vi "Drive Controller.vi"(8 "error in":errorcluster) -> ()   [LabVIEW 2020]
doc: "This VI executes continuously carrying out the current operation and responding to updates or new operation requests. It will often contain the timing or control code that is difficult to place directly in TeleOp. This VI generally opens all sensors and motors and isolates the rest of the robot code from knowing implementation details of how the operations are carried out."
uses:
  swerve/ctl/Pod Setpoints.ctl
  Drive Setpoints.ctl
  Drive Operations.ctl
  Robot Velocities.ctl
  <vilib>/Rock Robotics/WPI/ThirdParty/Phoenix-LabVIEW/Motor Controller/Controls/CTRE_Phoenix_MotorControl_ControlMode.ctl
  <vilib>/Analysis/coordinate.llb/Angle Range (Degree).ctl
  <vilib>/Analysis/coordinate.llb/Angle Units.ctl
  <vilib>/Analysis/coordinate.llb/Wrap Angle (array).vi
  <vilib>/Rock Robotics/Network Tables/NT Write Numeric Array.vi
  <vilib>/Analysis/NI_AAL_Angle.lvlib
panel:
  in  "Pod Setpoints (ft/s and deg)":T1
  out "CANCoder Angles":T2
  out "Calibration Error":errorcluster
  out "Initial Error":errorcluster
  out "Current\nCmd":string
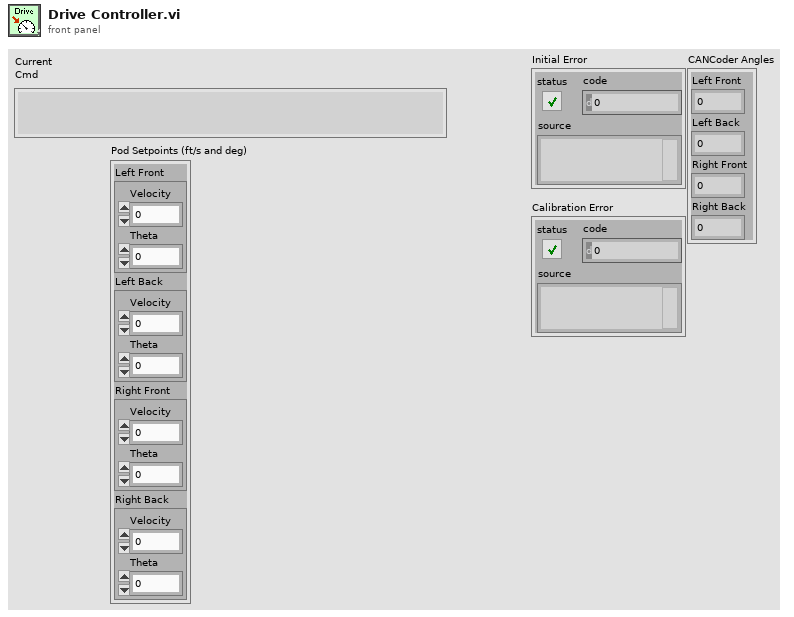
[diagram p1: front panel]
types:
  T1 = typedef "Pod Setpoints.ctl" = cluster{"Left Front":cluster{"Velocity":dbl, "Theta":dbl}, "Left Back":cluster{"Velocity":dbl, "Theta":dbl}, "Right Front":cluster{"Velocity":dbl, "Theta":dbl}, "Right Back":cluster{"Velocity":dbl, "Theta":dbl}}
  T2 = cluster{"Left Front":dbl, "Left Back":dbl, "Right Front":dbl, "Right Back":dbl}
  T3 = cluster{"LF radius":dbl[], "LB radius":dbl[], "RF radius":dbl[], "RB radius":dbl[]}
  T4 = cluster{"LF ID":u8, "LB ID":u8, "RF ID":u8, "RB ID":u8}
  T5 = typedef "Drive Setpoints.ctl" = cluster{"Operation":T6, "Robot Velocities":T7, "Field Centric?":bool, "Auto Velocities":T7[]}
  T6 = typedef "Drive Operations.ctl" = enum16{"Reserve", "Read Current", "Immediate", "Calibrate", "Reset Pods", "Auto"}
  T7 = typedef "Robot Velocities.ctl" = cluster{"vx":dbl, "vy":dbl, "w":dbl}
  T8 = typedef "Swerve Motors.ctl" = cluster{"Drive Motors":T9, "Steering Motors":T9}
  T9 = typedef "4 Motor Set.ctl" = cluster{"Left Front":T10, "Left Back":T10, "Right Front":T10, "Right Back":T10}
  T10 = typedef "WPI_MotorControlDeviceRef.ctl" = cluster{"DeviceStatus":errorcluster, "Type":T11, "PWM":cluster{"PWM Channel":T12, "DeadBand":T13}, "CAN":cluster{"Device Number":u8, "SetOutput VI Ref":variant, "GetOutput VI Ref":variant, "Enable VI Ref":variant, "Disable VI Ref":variant, "Data":variant}, "Invert":bool, "DIO PWM":cluster{"PWM \"Enable\" Channel":T12, "DIOChannel":T14, "PWM Rate":dbl}}
  T11 = typedef "WPI_MotorControlType.ctl" = enum16{"PWM", "CAN", "DIO PWM"}
  T12 = typedef "FPGA_DIOPWMChannel.ctl" = enum8{"PWM 0", "PWM 1", "PWM 2", "PWM 3", "PWM 4", "PWM 5", "PWM 6", "PWM 7", "PWM 8", "PWM 9", "PWM MXP 0", "PWM MXP 1", "PWM MXP 2", "PWM MXP 3", "PWM MXP 4", "PWM MXP 5", "PWM MXP 6", "PWM MXP 7", "PWM MXP 8", "PWM MXP 9", "Invalid"}
  T13 = typedef "WPI_PWMDeadband.ctl" = cluster{"Name":string, "maxPositivePwm":i32, "minPositivePwm":i32, "centerPwm":i32, "maxNegativePwm":i32, "minNegativePwm":i32, "angularRange":u16}
  T14 = typedef "FPGA_DIOChannel.ctl" = enum8{"DIO 0", "DIO 1", "DIO 2", "DIO 3", "DIO 4", "DIO 5", "DIO 6", "DIO 7", "DIO 8", "DIO 9", "DIO MXP 0", "DIO MXP 1", "DIO MXP 2", "DIO MXP 3", "DIO MXP 4", "DIO MXP 5", "DIO MXP 6", "DIO MXP 7", "DIO MXP 8", "DIO MXP 9", "DIO MXP 10", "DIO MXP 11", "DIO MXP 12", "DIO MXP 13", "DIO MXP 14", "DIO MXP 15", "SPI Port CS1", "SPI Port CS2", "SPI Port CS3", "SPI Port MISO", "SPI Port MOSI", "Invalid"}
  T15 = typedef "Swerve CANCoders.ctl" = cluster{"Left Front":T16, "Left Back":T16, "Right Front":T16, "Right Back":T16}
  T16 = typedef "CTRE_Phoenix_CANcoder_DeviceRef.ctl" = cluster{"DeviceStatus":errorcluster, "Device Number":u8, "Handle":u64, "UsageFrame":u32, "Library Path":path}
  T17 = typedef "Command Status Info.ctl" = cluster{"Name":string, "Status":T18, "notifier out":T19}
  T18 = typedef "Completion Status.ctl" = enum16{"Successful", "Aborted", "Incomplete"}
  T19 = typedef "Completion Notifier.ctl" = refnum<notifier>
  T20 = cluster{"SubSystem Data":T5, cluster{"Start Time (ms)":u32, "Iterations":i32}, cluster{"Command Info":T17, "Description":string, "Default Command":T5, "queue out":refnum<queue>, "Subsystem Name":string}}
  T21 = typedef "CTRE_PigeonIMU_DeviceRef.ctl" = cluster{"DeviceStatus":errorcluster, "Device Number":u8, "Type":T22, "Device ID":u32, "Handle":u64, "UsageFrame":u32, "Library Path":path}
  T22 = typedef "CTRE_PigeonIMU_ConnectionType.ctl" = u32
  T23 = typedef "CTRE_Phoenix_MotorControl_ControlMode.ctl" = u16
  T24 = cluster{"SubSystem Data":T5, cluster{"Start Time (ms)":u32, "Iterations":i32}, "Default Command Arguments":cluster{"Command Info":T17, "Description":string, "Default Command":T5, "queue out":refnum<queue>, "Subsystem Name":string}}
  T25 = typedef "NI_AAL_Angle.lvlib/Angle Units.ctl" = i32
  T26 = typedef "NI_AAL_Angle.lvlib/Angle Range (Degree).ctl" = u16
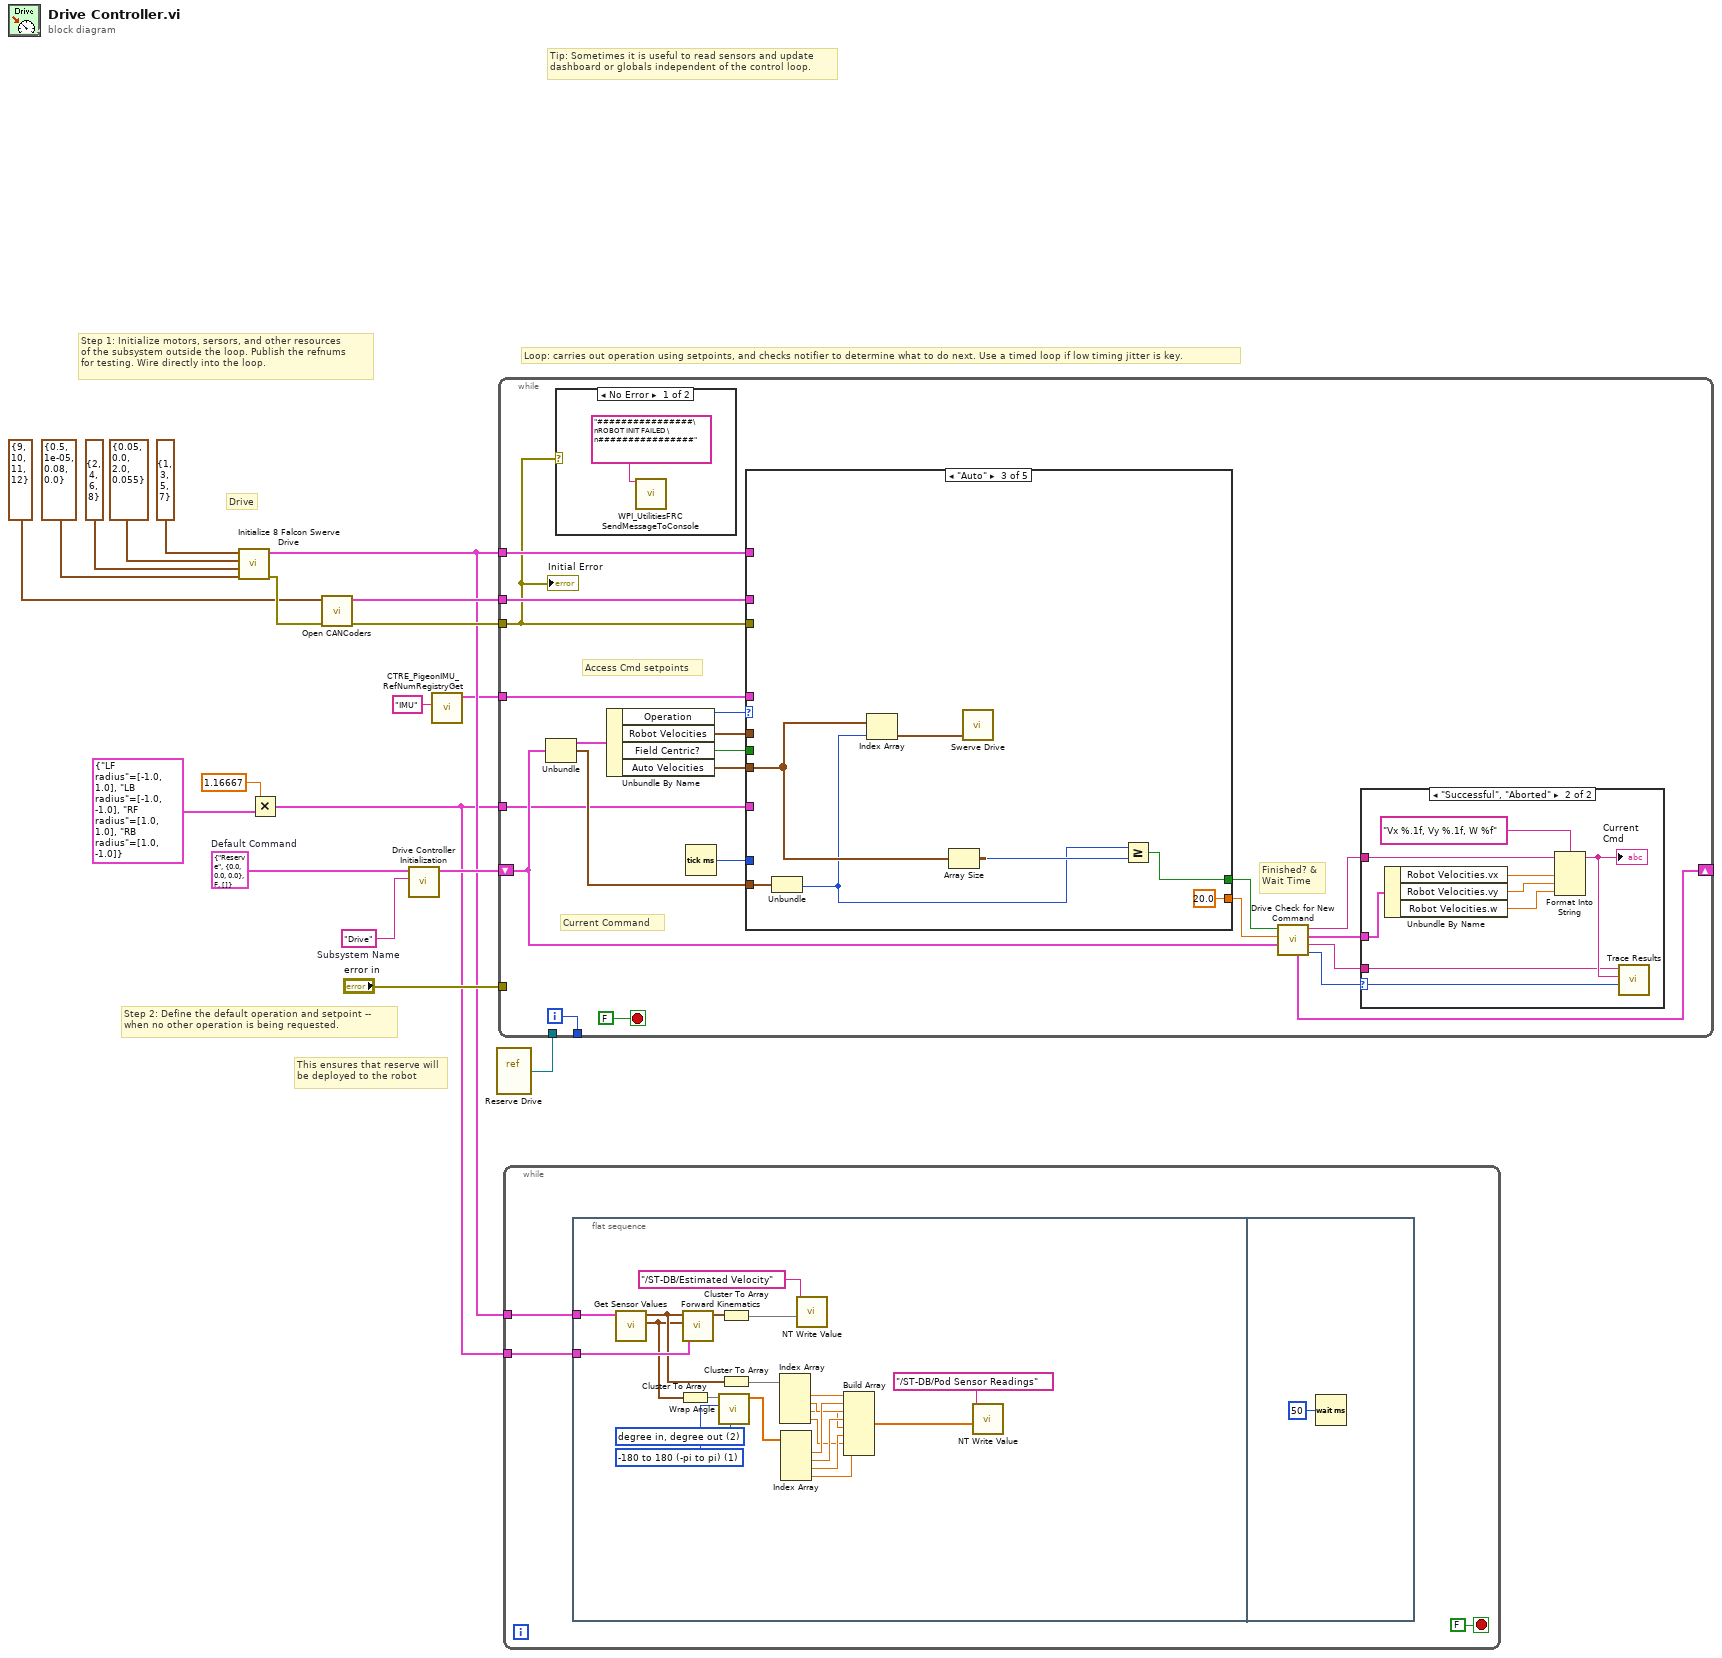
[diagram p0: block diagram]
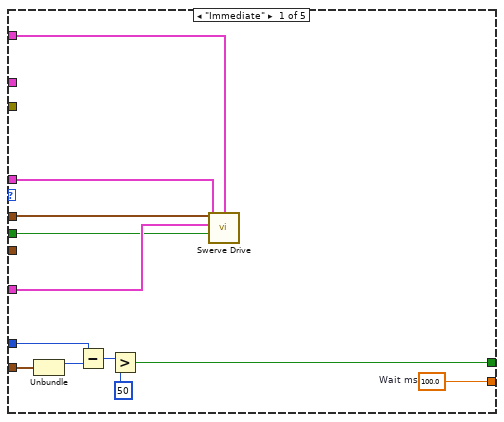
[diagram p4: hidden frame]
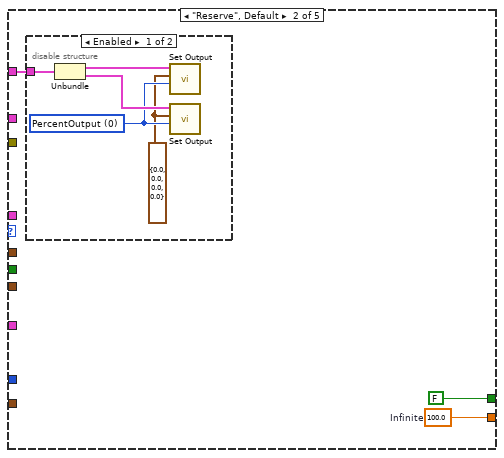
[diagram p5: hidden frame]
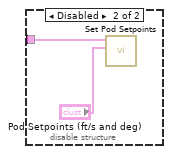
[diagram p6: hidden frame]
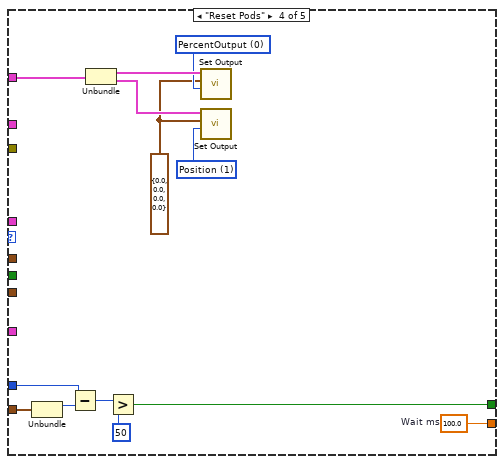
[diagram p7: hidden frame]
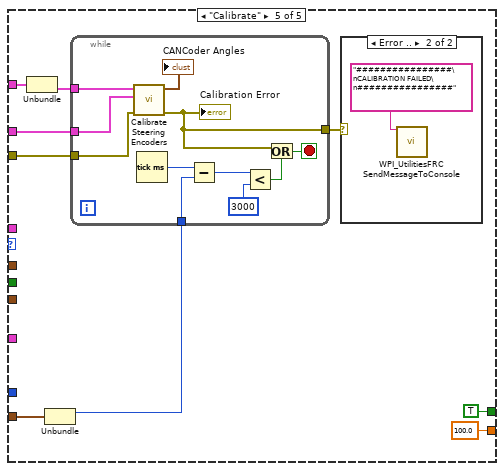
[diagram p8: hidden frame]
diagram:
  w15 = T5 {"Operation"=enum."Reserve", "Robot Velocities"={"vx"=0.0, "vy"=0.0, "w"=0.0}, "Field Centric?"=FALSE, "Auto Velocities"=[]}  # Default Command
  w19 = "Drive"  # Subsystem Name
  # "Drive"
  # "This ensures that reserve will\nbe deployed to the robot"
  # "Step 2: Define the default operation and setpoint --\nwhen no other operation is being requested."
  # "Step 1: Initialize motors, sersors, and other resources\nof the subsystem outside the loop. Publish the refnums\nfor testing. Wire directly into the loop."
  # "Loop: carries out operation using setpoints, and checks notifier to determine what to do next. Use a timed loop if low timing jitter is key."
  # "Tip: Sometimes it is useful to read sensors and update\ndashboard or globals independent of the control loop."
  n1 = call "Initialize 8 Falcon Swerve Drive.vi"("Steer PIDF"=cluster{"P":dbl, "I":dbl, "D":dbl, "F":dbl} {"P"=0.5, "I"=1e-05, "D"=0.08, "F"=0.0} ("PIDF"), "Steer CAN IDs"=T4 {"LF ID"=2, "LB ID"=4, "RF ID"=6, "RB ID"=8} ("Can IDs"), "Drive PIDF"=cluster{"P":dbl, "I":dbl, "D":dbl, "F":dbl} {"P"=0.05, "I"=0.0, "D"=2.0, "F"=0.055} ("PIDF"), "Drive CAN IDs"=T4 {"LF ID"=1, "LB ID"=3, "RF ID"=5, "RB ID"=7} ("Can IDs")) -> ("error out"=w10:errorcluster, "Motors"=w4:T8)  [unwired: 6 in]
  n2 = Multiply(x=1.16667, y=T3 {"LF radius"=[-1.0, 1.0], "LB radius"=[-1.0, -1.0], "RF radius"=[1.0, 1.0], "RB radius"=[1.0, -1.0]} ("Radii")) -> (x*y=w3:T3)
  n3 = call "Open CANCoders.vi"("error in"=w10, "CANCoder Can IDs"=T4 {"LF ID"=9, "LB ID"=10, "RF ID"=11, "RB ID"=12}) -> ("error out"=w7:errorcluster, "CANCoders"=w8:T15)  [unwired: 8 in]
  n4 = call "Drive Controller Initialization.vi"("Subsystem Name"=w19, "Default Command"=w15) -> ("Current Command"=w17:T20)  [unwired: 9 in]
  n5 = call <vilib>:"CTRE_PigeonIMU_RefNumRegistryGet.vi"("refnum name"="IMU") -> ("PigeonIMUDevRef"=w1:T21)  [unwired: 9 in, 1 out]
  n6 = vi-ref "Reserve Drive.vi"() -> (w16:refnum<vi>)
  n7 = while {
    shift-right: [w35] -> _
    shift-left: w17 -> [w28]
    tunnel: [w40] -> _
    tunnel: "error in" -> [_]
    tunnel: w16 -> [_]
    tunnel: w4 -> [w23]
    tunnel: w8 -> [w26]
    tunnel: w7 -> [w22]
    tunnel: w3 -> [w24]
    tunnel: w1 -> [w21]
    i -> [w40]
    stop <- FALSE stop-if-true
    # "Current Command"
    # "Access Cmd setpoints"
    # "Finished? &\nWait Time"
    n8 = Unbundle(w28) -> ("SubSystem Data"=w39:T5, w29:cluster{"Start Time (ms)":u32, "Iterations":i32})  [unwired: 1 out]
    n9 = case shown="No Error" w22 {
      frame No Error {
        n10 = call <vilib>:"WPI_UtilitiesFRC SendMessageToConsole.vi"("Message"="################\nROBOT INIT FAILED \n################") -> ()  [unwired: 14 in, 1 out]
      }
      frame Error {
      }
    }
    n11 = Unbundle By Name(w39) -> ("Operation"=w38:T6, "Robot Velocities"=w27:T7, "Field Centric?"=w25:bool, "Auto Velocities"=w20:T7[])
    n12 = Tick Count (ms)() -> (millisecond timer value=w37:u32)
    n13 = case shown="\"Auto\"" w38 {
      tunnel: [w63 w66 20.0 ("Infinite") w81 100.0 ("Infinite")] -> w34
      tunnel: [w55 FALSE ("ignore previous (F)") w75 w82 TRUE ("ignore previous (F)")] -> w33
      tunnel: w29 -> [w60 _ w80 w83 w96]
      tunnel: w37 -> [w59 _ _ w84 _]
      tunnel: w27 -> [w52 _ _ _ _]
      tunnel: w23 -> [w61 w64 _ w90 w99]
      tunnel: w26 -> [_ _ _ _ w102]
      tunnel: w22 -> [_ _ _ _ w100]
      tunnel: w25 -> [w54 _ _ _ _]
      tunnel: w24 -> [w62 _ _ _ _]
      tunnel: w21 -> [w53 _ _ _ _]
      tunnel: w20 -> [_ _ w77 _ _]
      frame "Immediate" {
        w63 = 100.0  # Wait ms
        n14 = Unbundle(w60) -> ("Start Time (ms)"=w58:u32)  [unwired: 1 out]
        n15 = Subtract(x=w59, y=w58) -> (x-y=w57:u32)
        n16 = Greater?(x=w57, y=u32 50) -> (0:w55:bool)
        n17 = call "Swerve Drive.vi"("Field Centric?"=w54, "Cluster"=w62, "Robot Velocities"=w52, "PigeonIMUDevRef"=w53, "Motors"=w61) -> ()  [unwired: 7 in]
      }
      frame "Reserve", Default {
        w66 = 100.0  # Infinite
        n18 = disable-structure shown="Enabled" {
          disable-tunnel: w64 -> [w71 w73]
          frame Enabled {
            w68 = T23 0 items=["PercentOutput"=0, "Position"=1, "Velocity"=2, "Current"=3, "Follower"=5, "MotionProfile"=6, "MotionMagic"=7, "MotionProfileArc"=10, "Disabled"=15] ("Control Mode")
            w67 = T2 {"Left Front"=0.0, "Left Back"=0.0, "Right Front"=0.0, "Right Back"=0.0} ("Setpoints")
            n19 = Unbundle(w71) -> ("Drive Motors"=w69:T9, "Steering Motors"=w70:T9)
            n20 = call "Set Output.vi"("Control Mode"=w68, "Setpoints"=w67, "Motors"=w69) -> ()  [unwired: 9 in]
            n21 = call "Set Output.vi"("Control Mode"=w68, "Setpoints"=w67, "Motors"=w70) -> ()  [unwired: 9 in]
          }
          frame Disabled {
            n22 = call "Set Pod Setpoints.vi"("Pod Setpoints (ft/s and deg)"="Pod Setpoints (ft/s and deg)", "Motors"=w73) -> ()  [unwired: 10 in]
          }
        }
      }
      frame "Auto" {
        n23 = Unbundle(w80) -> ("Iterations"=w74:i32)  [unwired: 1 out]
        n24 = Index Array(array=w77, index=w74) -> (element=w79:T7)
        n25 = Array Size(array=w77) -> (size(s)=w76:i32)
        n26 = call "Swerve Drive.vi"("Robot Velocities"=w79) -> ()  [unwired: 11 in]
        n27 = Greater Or Equal?(x=w74, y=w76) -> (x >= y?=w75:bool)
      }
      frame "Reset Pods" {
        w81 = 100.0  # Wait ms
        w88 = T2 {"Left Front"=0.0, "Left Back"=0.0, "Right Front"=0.0, "Right Back"=0.0} ("Setpoints")
        w89 = T23 0 items=["PercentOutput"=0, "Position"=1, "Velocity"=2, "Current"=3, "Follower"=5, "MotionProfile"=6, "MotionMagic"=7, "MotionProfileArc"=10, "Disabled"=15] ("Control Mode")
        w91 = T23 1 items=["PercentOutput"=0, "Position"=1, "Velocity"=2, "Current"=3, "Follower"=5, "MotionProfile"=6, "MotionMagic"=7, "MotionProfileArc"=10, "Disabled"=15] ("Control Mode")
        n28 = Unbundle(w83) -> ("Start Time (ms)"=w87:u32)  [unwired: 1 out]
        n29 = Subtract(x=w84, y=w87) -> (x-y=w86:u32)
        n30 = Unbundle(w90) -> ("Drive Motors"=w92:T9, "Steering Motors"=w93:T9)
        n31 = Greater?(x=w86, y=u32 50) -> (0:w82:bool)
        n32 = call "Set Output.vi"("Control Mode"=w89, "Setpoints"=w88, "Motors"=w92) -> ()  [unwired: 9 in]
        n33 = call "Set Output.vi"("Control Mode"=w91, "Setpoints"=w88, "Motors"=w93) -> ()  [unwired: 9 in]
      }
      frame "Calibrate" {
        n34 = Unbundle(w99) -> ("Steering Motors"=w98:T9)  [unwired: 1 out]
        n35 = Unbundle(w96) -> ("Start Time (ms)"=w95:u32)  [unwired: 1 out]
        n36 = while {
          tunnel: w102 -> [w114]
          tunnel: w100 -> [w113]
          tunnel: w98 -> [w112]
          tunnel: w95 -> [w109]
          tunnel: [w104] -> w94
          stop <- w110 stop-if-true
          n37 = call "Calibrate Steering Encoders.vi"("error in"=w113, "CANCoders"=w114, "Steering Motors"=w112) -> ("error out"=w104:errorcluster, "CANCoder Angles"=→"CANCoder Angles":T2)  [unwired: 7 in]
          "Calibration Error" <- w104
          n38 = Tick Count (ms)() -> (millisecond timer value=w108:u32)
          n39 = Subtract(x=w108, y=w109) -> (x-y=w107:u32)
          n40 = Less?(x=w107, y=u32 3000) -> (x < y?=w105:bool)
          n41 = Or(x=w104, y=w105) -> (x .or. y?=w110:bool)
        }
        n42 = case shown="Error .." w94 {
          frame No Error {
          }
          frame Error {
            n43 = call <vilib>:"WPI_UtilitiesFRC SendMessageToConsole.vi"("Message"="################\nCALIBRATION FAILED\n################") -> ()  [unwired: 14 in, 1 out]
          }
        }
      }
    }
    n44 = call "Drive Check for New Command.vi"("input cluster"=w28, "Wait time (ms)"=w34, "Finished?"=w33) -> ("Completion"=w36:T18, "Subsystem Name"=w30:string, "Current Command"=w31:T5, "Initial Trace String"=w32:string, "Next Command"=w35:T24)  [unwired: 4 in]
    n45 = case shown="\"Successful\", \"Aborted\"" w36 {
      selector: w36 -> [_ w51]
      tunnel: w32 -> [_ w46]
      tunnel: w31 -> [_ w47]
      tunnel: w30 -> [_ w43]
      frame "Incomplete", Default {
        # "Continuing current command"
      }
      frame "Successful", "Aborted" {
        # "Report and setup for next command"
        n46 = Unbundle By Name(w47) -> ("Robot Velocities.vx"=w49:dbl, "Robot Velocities.vy"=w50:dbl, "Robot Velocities.w"=w44:dbl)
        n47 = Format Into String(format string="Vx %.1f, Vy %.1f, W %f", initial string=w46, w49, w50, w44) -> (resulting string=w45:string)  [unwired: 1 in, 1 out]
        "Current\nCmd" <- w45
        n48 = call <vilib>:"Trace Results.vi"("Status of previous command"=w51, "Description"=w45, "Subsystem"=w43) -> ()  [unwired: 9 in]
      }
    }
    "Initial Error" <- w22
  }
  n49 = while {
    tunnel: w4 -> [w117]
    tunnel: w3 -> [w115]
    stop <- FALSE stop-if-true
    n50 = flat-sequence {
      tunnel: w117 -> [w139]
      tunnel: w115 -> [w138]
      frame #0 {
        w118 = T25 2 items=["radian in, radian out", "radian in, degree out", "degree in, degree out", "degree in, radian out"] ("angle units")
        w119 = T26 1 items=["none", "-180 to 180 (-pi to pi)", "0 to 360 (0 to 2pi)"] ("angle range")
        n51 = call "Get Sensor Values.vi"("Motors"=w139) -> ("Steer Angles (degrees)"=w122:T2, "Drive Velocities (ft/s)"=w133:T2)  [unwired: 7 in, 2 out]
        n52 = Cluster To Array(cluster=w122) -> (array=w121:dbl[])
        n53 = call "Forward Kinematics.vi"("Radii (ft)"=w138, "Steer Angles (degrees)"=w122, "Drive Velocities (ft/s)"=w133) -> ("Robot Velocities (ft and deg)/s"=w137:cluster{"vx":dbl, "vy":dbl, "w":dbl})  [unwired: 8 in]
        n54 = call-poly <vilib>:"Wrap Angle.vi"("angle units"=w118, "angle range"=w119, "Angle In"=w121) -> ("Angle Out"=w120:dbl[])  [unwired: 7 in, 1 out]
        n55 = Cluster To Array(cluster=w137) -> (array=w136:dbl[])
        n56 = Cluster To Array(cluster=w133) -> (array=w134:dbl[])
        n57 = Index Array(array=w134) -> (element #1=w131:dbl, element #2=w129:dbl, element #3=w127:dbl, element #4=w125:dbl)  [unwired: 4 in]
        n58 = Index Array(array=w120) -> (element #1=w130:dbl, element #2=w128:dbl, element #3=w126:dbl, element #4=w124:dbl)  [unwired: 4 in]
        n59 = call-poly <vilib>:"NT Write Value.vi"("Numeric Array"=w136, "Name"="/ST-DB/Estimated Velocity") -> ()  [unwired: 9 in, 1 out]
        n60 = Build Array(w131, w130, w129, w128, w127, w126, w125, w124) -> (w123:dbl[])
        n61 = call-poly <vilib>:"NT Write Value.vi"("Numeric Array"=w123, "Name"="/ST-DB/Pod Sensor Readings") -> ()  [unwired: 9 in, 1 out]
      }
      frame #1 {
        n62 = Wait (ms)(milliseconds to wait=u32 50) -> ()  [unwired: 1 out]
      }
    }
  }
